vi "Simple Event Handler.vi"(11 "Error In":errorcluster) -> (15 "Error Out":errorcluster)   [LabVIEW 2020]
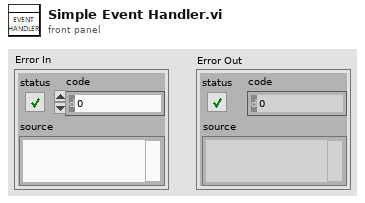
[diagram p1: front panel]
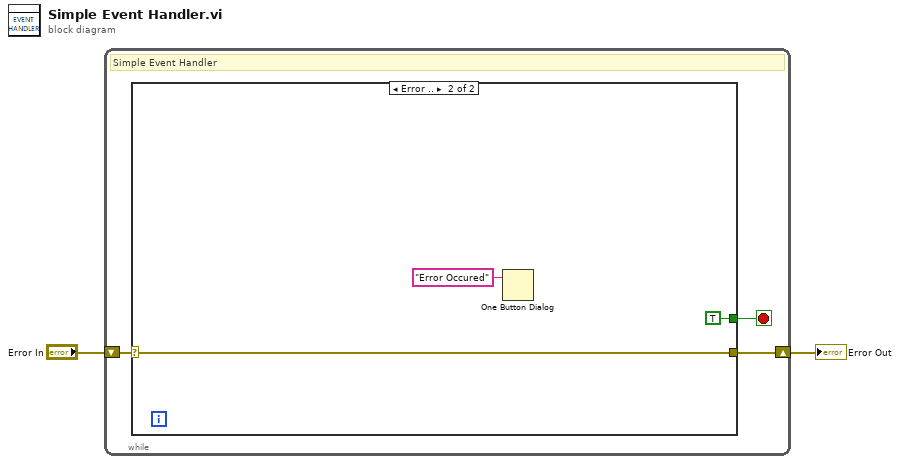
[diagram p0: block diagram]
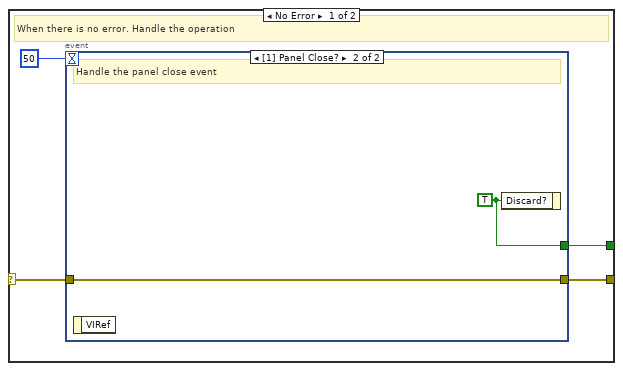
[diagram p2: hidden frame]
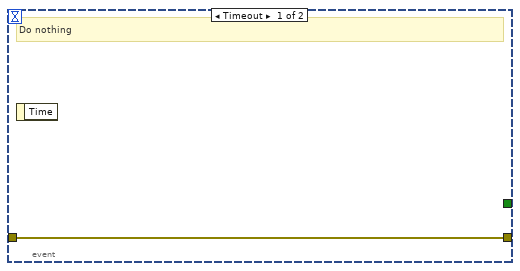
[diagram p3: hidden frame]
diagram:
  n1 = while {
    shift-right: [w4] -> w1
    shift-left: "Error In" -> [w5]
    stop <- w3 stop-if-true
    # "Simple Event Handler"
    n2 = case shown="Error .." w5 {
      selector: w5 -> [w8 w15]
      tunnel: [w7 w15] -> w4
      tunnel: [w6 TRUE ("Discard?")] -> w3
      frame No Error {
        # "When there is no error. Handle the operation"
        n3 = event shown="[1] Panel Close?" {
          selector: _ -> [_ _]
          dyn-events: _ -> [_ _]
          timeout: 50 -> [_ _]
          tunnel: [w10 w12] -> w7
          tunnel: w8 -> [w10 w12]
          tunnel: [_ w11] -> w6
          event Timeout {
            # "Do nothing"
            n4 = event-data() -> ()  [unwired: 1 in, 1 out]
          }
          event Panel Close? {
            w11 = TRUE ("Discard?")
            # "Handle the panel close event"
            n5 = event-data() -> ()  [unwired: 1 in, 1 out]
            n6 = event-data("Discard?"=w11) -> ()  [unwired: 1 in, 1 out]
          }
        }
      }
      frame Error {
        n7 = One Button Dialog(message="Error Occured") -> ()  [unwired: 1 in, 1 out]
      }
    }
  }
  "Error Out" <- w1
